vi "CSGaussmeter.add services.vi"(0 "i ref in":refnum<vi>, 5 "ms timeout (10000)":i32=10000, 7 "Name":string, 9 "VISA Resource Name":refnum<visa-resource-name>, 11 "error in (no error)":errorcluster) -> (4 "i ref out":refnum<vi>, 8 "timed out":bool, 15 "error out":errorcluster)   [LabVIEW 2014, in "CSGaussmeter.lvlib"]
uses:
  CSGaussmeter.lvlib
  CS_Core/CSSystem/CSSystemLib/CSSystemLib.lvlib
  CSlibraries-extern/DimLVEvent/LVDimInterface/LVDimInterface.lvlib
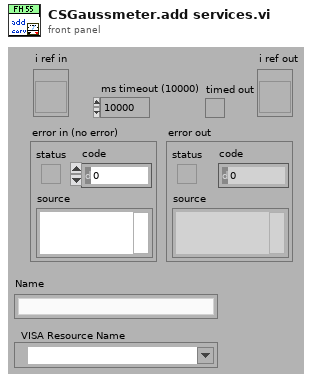
[diagram p1: front panel]
types:
  T1 = typedef "CSGaussmeter.lvlib/CSGaussmeter.i attribute.ctl" = cluster{"Name":string, "VISA Resource Name":refnum<visa-resource-name>, "actValues":cluster{" Limit":bool, "Unit ":T2, "Temp_Unit":T3, "Max":T4, " Filter":bool, " Peak":bool, " Auto_Range":bool, "Range":T5, " Rel":bool, " CTemp":bool, " CField":bool, "AC_DC ":bool, "Set_lower":cluster{"Numeric":dbl, "Cancel Button":bool, "Unit":T6}, "Set_upper":cluster{"Numeric":dbl, "Cancel Button":bool, "Unit":T6}, "Set_Rel":cluster{"Numeric":dbl, "Cancel Button":bool, "Unit":T6}, "Zero":bool, " Local":bool, "Reset":bool, " Init":bool}, "FH 55 Gauss-/Teslameter":T7, "MAX_Value":T8, "MIN_Value":T8, "Rel_Value":T8, "Array ":string[], "LIMU":dbl, " LIML":dbl, "Messwerte 2":string, "Messwerte ":cluster{"Numeric":i32, "OK Button":bool}, "serviceID":cluster{"Current ID":i32, "Unit ID":i32, "Temp ID":i32, "Name ID \n":i32, "Visa ID ":i32}, "setValues ":cluster{" Limit":bool, "Unit ":T2, "Temp_Unit":T3, "Max":T4, " Filter":bool, " Peak":bool, " Auto_Range":bool, "Range":T5, " Rel":bool, " CTemp":bool, " CField":bool, "AC_DC ":bool, "Set_lower":cluster{"Numeric":dbl, "Cancel Button":bool, "Unit":T6}, "Set_upper":cluster{"Numeric":dbl, "Cancel Button":bool, "Unit":T6}, "Set_Rel":cluster{"Numeric":dbl, "Cancel Button":bool, "Unit":T6}, "Zero":bool, " Local":bool, "Reset":bool, " Init":bool}}
  T2 = typedef "FH 55.lvlib/Unit.ctl" = enum16{"T", "G", "A/m"}
  T3 = typedef "FH 55.lvlib/Temp_Unit.ctl" = enum16{"Temp off", "Celsius", "Fahrenheit"}
  T4 = typedef "FH 55.lvlib/Max.ctl" = enum16{"MAX off", "Show MAX", "MAX/MIN"}
  T5 = typedef "FH 55.lvlib/Range.ctl" = enum16{"1", "2", "3", "4", "5", "6", "7"}
  T6 = typedef "FH 55.lvlib/Unit2.ctl" = enum16{"mT", "G", "kA/m"}
  T7 = typedef "FH 55.lvlib/Display.ctl" = cluster{"current value":string, "Limit":string, "Remote":string, "function ":string, "Cluster":cluster{"AC/DC":string, "Auto":string, "Filter":string, "Range":string, "Rel":string, "Peak":string}}
  T8 = typedef "FH 55.lvlib/Value_String.ctl" = cluster{"Numeric":dbl, "String":string}
  T9 = cluster{"Current ID":i32, "Unit ID":i32, "Temp ID":i32, "Name ID \n":i32, "Visa ID ":i32}
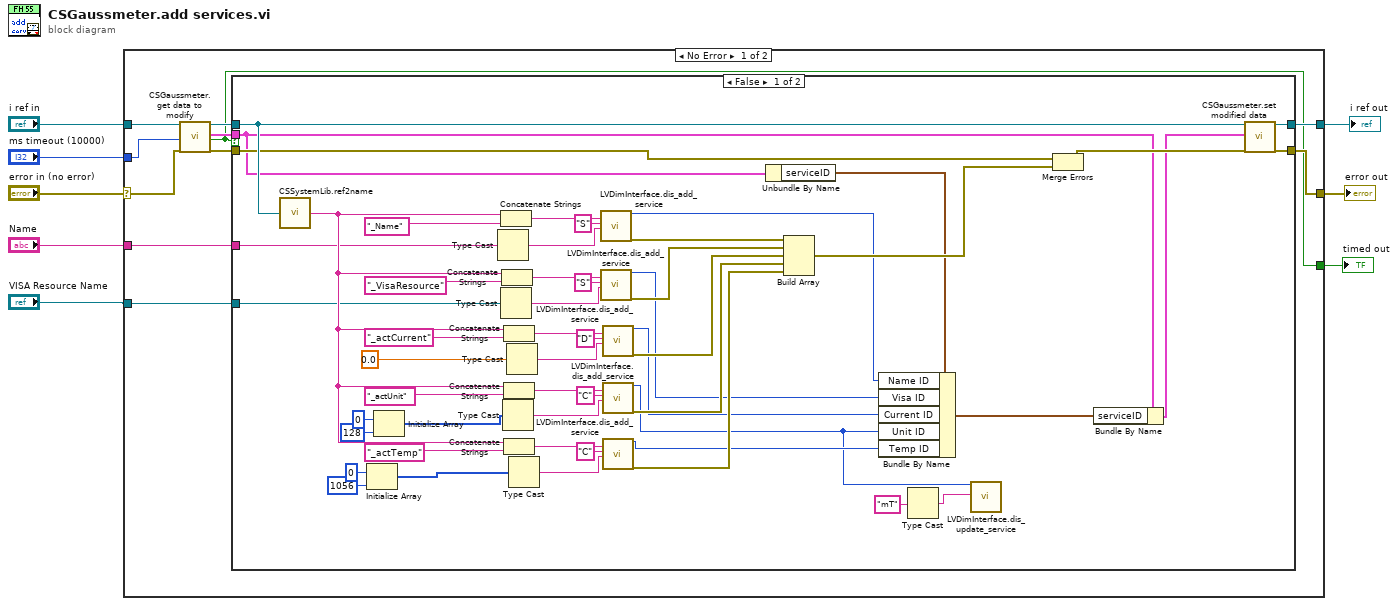
[diagram p0: block diagram]
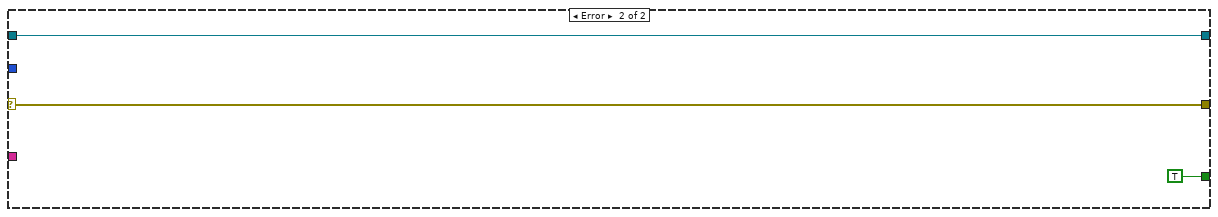
[diagram p3: hidden frame]
diagram:
  n1 = case shown="No Error" "error in (no error)" {
    selector: "error in (no error)" -> [w11 w75]
    tunnel: "ms timeout (10000)" -> [w19 _]
    tunnel: "i ref in" -> [w18 w76]
    tunnel: [w14 w76] -> w4
    tunnel: [w13 w75] -> w3
    tunnel: [w12 TRUE ("timed out")] -> w2
    tunnel: "Name" -> [w10 _]
    tunnel: "VISA Resource Name" -> [w9 _]
    frame No Error {
      n2 = call "CSGaussmeter.get data to modify.vi"("i ref in"=w18, "ms timeout (10000)"=w19, "error in (no error)"=w11) -> ("i ref out"=w16:refnum<vi>, "i attribute"=w17:T1, "timed out"=w12:bool, "error out"=w15:errorcluster)  [unwired: 13 in]
      n3 = case shown="False" w12 {
        tunnel: w17 -> [w35 _]
        tunnel: w16 -> [w70 w73]
        tunnel: w15 -> [w52 w72]
        tunnel: [w71 w73] -> w14
        tunnel: [w69 w72] -> w13
        tunnel: w10 -> [w37 _]
        tunnel: w9 -> [w38 _]
        frame False {
          n4 = call "CSSystemLib.ref2name.vi"("obj refnum"=w70) -> ("name"=w41:string)
          n5 = Initialize Array(i8 0, 1056 ("dimension size")) -> (w23:i8[])
          n6 = Initialize Array(i8 0, 128 ("dimension size")) -> (w26:i8[])
          n7 = Type Cast(x=w37) -> (*(type *) &x=w43:string)  [unwired: 1 in]
          n8 = Concatenate Strings(w41, "_Name") -> (w42:string)
          n9 = Type Cast(x=w38) -> (*(type *) &x=w47:string)  [unwired: 1 in]
          n10 = Concatenate Strings(w41, "_VisaResource") -> (w44:string)
          n11 = Type Cast(x=w26) -> (*(type *) &x=w62:string)  [unwired: 1 in]
          n12 = Concatenate Strings(w41, "_actCurrent") -> (w65:string)
          n13 = Concatenate Strings(w41, "_actUnit") -> (w63:string)
          n14 = Concatenate Strings(w41, "_actTemp") -> (w61:string)
          n15 = Type Cast(x=0.0 ("D32")) -> (*(type *) &x=w64:string)  [unwired: 1 in]
          n16 = Type Cast(x=w23) -> (*(type *) &x=w60:string)  [unwired: 1 in]
          n17 = call "LVDimInterface.dis_add_service.vi"("serviceName"=w42, "typeDescriptor"="S", "data"=w43) -> ("my_serviceID"=w32:i32, "error out"=w39:errorcluster)  [unwired: 15 in]
          n18 = call "LVDimInterface.dis_add_service.vi"("serviceName"=w44, "typeDescriptor"="S", "data"=w47) -> ("my_serviceID"=w33:i32, "error out"=w40:errorcluster)  [unwired: 15 in]
          n19 = call "LVDimInterface.dis_add_service.vi"("serviceName"=w65, "typeDescriptor"="D", "data"=w64) -> ("my_serviceID"=w36:i32, "error out"=w56:errorcluster)  [unwired: 15 in]
          n20 = call "LVDimInterface.dis_add_service.vi"("serviceName"=w63, "typeDescriptor"="C", "data"=w62) -> ("my_serviceID"=w22:i32, "error out"=w55:errorcluster)  [unwired: 15 in]
          n21 = call "LVDimInterface.dis_add_service.vi"("serviceName"=w61, "typeDescriptor"="C", "data"=w60) -> ("my_serviceID"=w29:i32, "error out"=w54:errorcluster)  [unwired: 15 in]
          n22 = Unbundle By Name(w35) -> ("serviceID"=w34:T9)
          n23 = Build Array(w39, w40, w56, w55, w54) -> (w53:errorcluster[])
          n24 = Bundle By Name(cluster=w34, "Name ID"=w32, "Visa ID"=w33, "Current ID"=w36, "Unit ID"=w22, "Temp ID"=w29) -> (w31:T9)
          n25 = Type Cast(x="mT") -> (*(type *) &x=w21:string)  [unwired: 1 in]
          n26 = call "LVDimInterface.dis_update_service.vi"("my_serviceID"=w22, "data"=w21) -> ()  [unwired: 15 in, 3 out]
          n27 = Merge Errors(w52, w53) -> (w51:errorcluster)
          n28 = Bundle By Name(cluster=w35, "serviceID"=w31) -> (w30:T1)
          n29 = call "CSGaussmeter.set modified data.vi"("i ref in"=w70, "i attribute"=w30, "error in (no error)"=w51) -> ("i ref out"=w71:refnum<vi>, "error out"=w69:errorcluster)  [unwired: 15 in]
        }
        frame True {
        }
      }
    }
    frame Error {
    }
  }
  "error out" <- w3
  "i ref out" <- w4
  "timed out" <- w2
